vi "Get Type.vi"(11 "StringPanel in":refnum<class "StringPanel.lvclass">) -> (2 "Type":refnum<class "Type.lvclass">)   [LabVIEW 2020, in "Conditum-Tools.lvlib" / "StringPanel.lvclass"]
uses:
  StringPanel.lvclass
  Conditum-Clone/Columns/Type/Type.lvclass
  StringPanel.lvclass/StringPanel.ctl
  Conditum-Clone/Columns/String/String.lvclass
  C:/dev/lv20CE/lv-conditum-tools/Conditum-Clone/Columns/Type/Type.lvclass
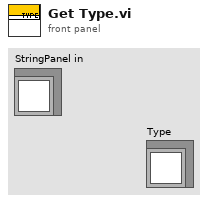
[diagram p1: front panel]
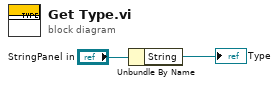
[diagram p0: block diagram]
diagram:
  n1 = Unbundle By Name("StringPanel in") -> ("String"=→"Type":refnum<class "String.lvclass">)
